vi "MessageName.vi"() -> (2 "MessageName":string)   [LabVIEW 2020, in "ReplyOneDouble.lvlib"]
uses:
  ReplyOneDouble.lvlib
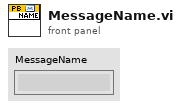
[diagram p1: front panel]
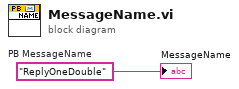
[diagram p0: block diagram]
diagram:
  w1 = "ReplyOneDouble"  # PB MessageName
  "MessageName" <- w1
